vi "Configure Measurement (Power Stat CCDF).vi"(0 "VISA resource name":refnum<visa-resource-name>, 1 "Information Bandwidth (5E+6 Hz)":dbl=5000000.0, 5 "Sampling Points (1E+7)":i32=10000000 format="%.0g", 7 "Measurement Cycles (1)":i32=1 format="%.0g", 9 "Measurement Interval (0.001 s)":dbl=0.001, 11 "error in (no error)":errorcluster) -> (4 "VISA resource name out":refnum<visa-resource-name>, 15 "error out":errorcluster)   [LabVIEW 2014, in "Agilent MXA Series.lvlib"]
doc: "Sets the Power Stat CCDF measurement parameters."
uses:
  Agilent MXA Series.lvlib
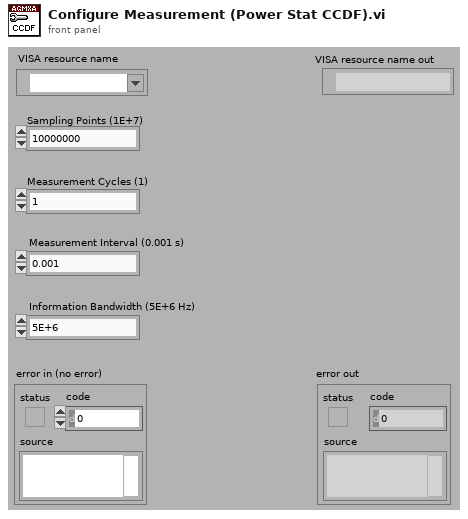
[diagram p1: front panel]
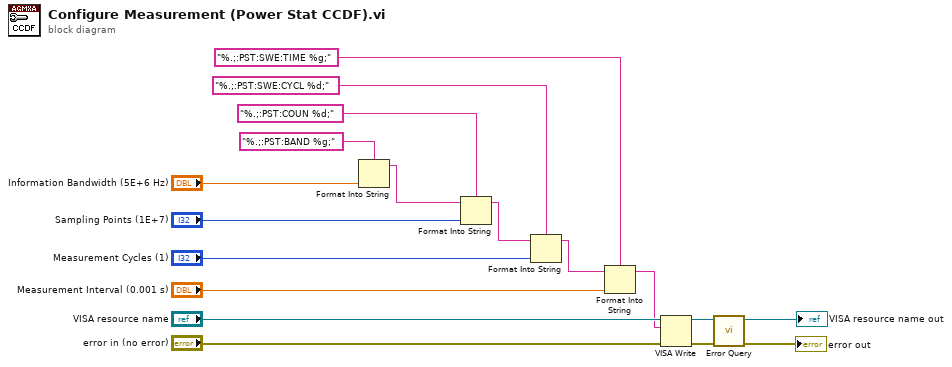
[diagram p0: block diagram]
diagram:
  n1 = Format Into String(format string="%.;:PST:BAND %g;", "Information Bandwidth (5E+6 Hz)") -> (resulting string=w15:string)  [unwired: 2 in, 1 out]
  n2 = Format Into String(format string="%.;:PST:COUN %d;", initial string=w15, "Sampling Points (1E+7)") -> (resulting string=w11:string)  [unwired: 1 in, 1 out]
  n3 = Format Into String(format string="%.;:PST:SWE:CYCL %d;", initial string=w11, "Measurement Cycles (1)") -> (resulting string=w8:string)  [unwired: 1 in, 1 out]
  n4 = Format Into String(format string="%.;:PST:SWE:TIME %g;", initial string=w8, "Measurement Interval (0.001 s)") -> (resulting string=w5:string)  [unwired: 1 in, 1 out]
  n5 = VISA Write(VISA resource name="VISA resource name", write buffer=w5, error in (no error)="error in (no error)") -> (VISA resource name out=w3:refnum<visa-resource-name>, error out=w4:errorcluster)  [unwired: 1 out]
  n6 = call "Error Query.vi"("error in (no error)"=w4, "VISA resource name"=w3) -> ("error out"=→"error out":errorcluster, "VISA resource name out"=→"VISA resource name out":refnum<visa-resource-name>)  [unwired: 6 in, 2 out]
